vi "use item msg.vi"(9 "P1 turn":bool, 10 "Item num":u32) -> (2 "String":string)   [LabVIEW 2025]
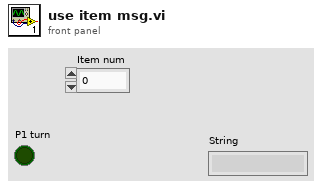
[diagram p1: front panel]
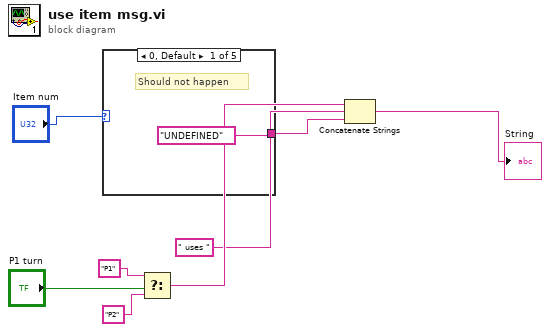
[diagram p0: block diagram]
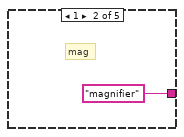
[diagram p2: hidden frame]
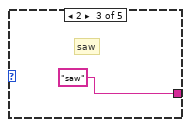
[diagram p3: hidden frame]
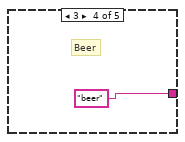
[diagram p4: hidden frame]
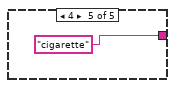
[diagram p5: hidden frame]
diagram:
  n1 = case shown="0, Default" "Item num" {
    tunnel: ["UNDEFINED" "magnifier" "saw" "beer" "cigarette"] -> w2
    frame 0, Default {
      # "Should not happen"
    }
    frame 1 {
      # "mag"
    }
    frame 2 {
      # "saw"
    }
    frame 3 {
      # "Beer"
    }
    frame 4 {
    }
  }
  n2 = Select(t="P1", s="P1 turn", f="P2") -> (s? t:f=w5:string)
  n3 = Concatenate Strings(w5, " uses ", w2) -> (→"String":string)
